vi "Read CarWash Controller Constants.vi"(8 "error in":errorcluster, 11 "CFG File Refnum in":T2) -> (0 "error out":errorcluster, 3 "CFG File Refnum out":T2)   [LabVIEW 2017]
uses:
  <vilib>/Utility/config.llb/Config Data RefNum.ctl
  Configuration Data.ctl
  Car Wash System Globals.vi
  <vilib>/Utility/config.llb/Read Key (U32).vi
  <vilib>/Utility/error.llb/Error Cluster From Error Code.vi
  <vilib>/ErrorRing/Error Ring.xnode
  <vilib>/Utility/config.llb/NI_LVConfig.lvlib
panel:
  out "Cluster":T1
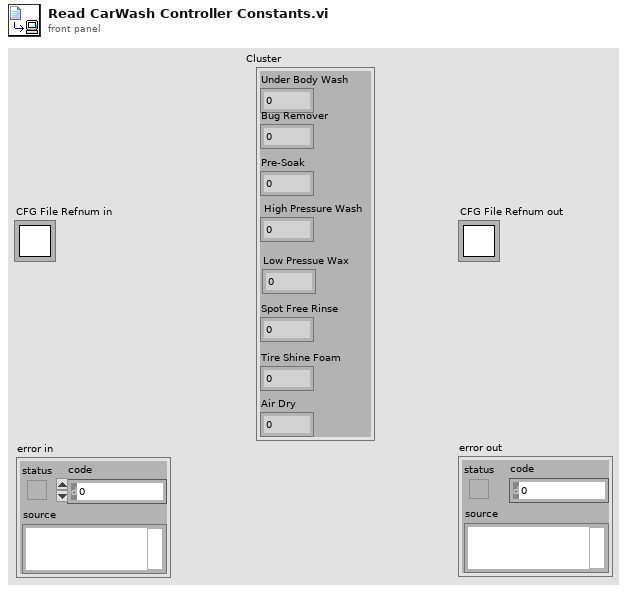
[diagram p1: front panel]
types:
  T1 = typedef "Configuration Data.ctl" = cluster{"Under Body Wash ":u32, "Bug Remover":u32, "Pre-Soak":u32, " High Pressure Wash":u32, "Low Pressue Wax ":u32, "Spot Free Rinse ":u32, "Tire Shine Foam":u32, "Air Dry ":u32}
  T2 = typedef "NI_LVConfig.lvlib/Config Data RefNum.ctl" = refnum<k1>
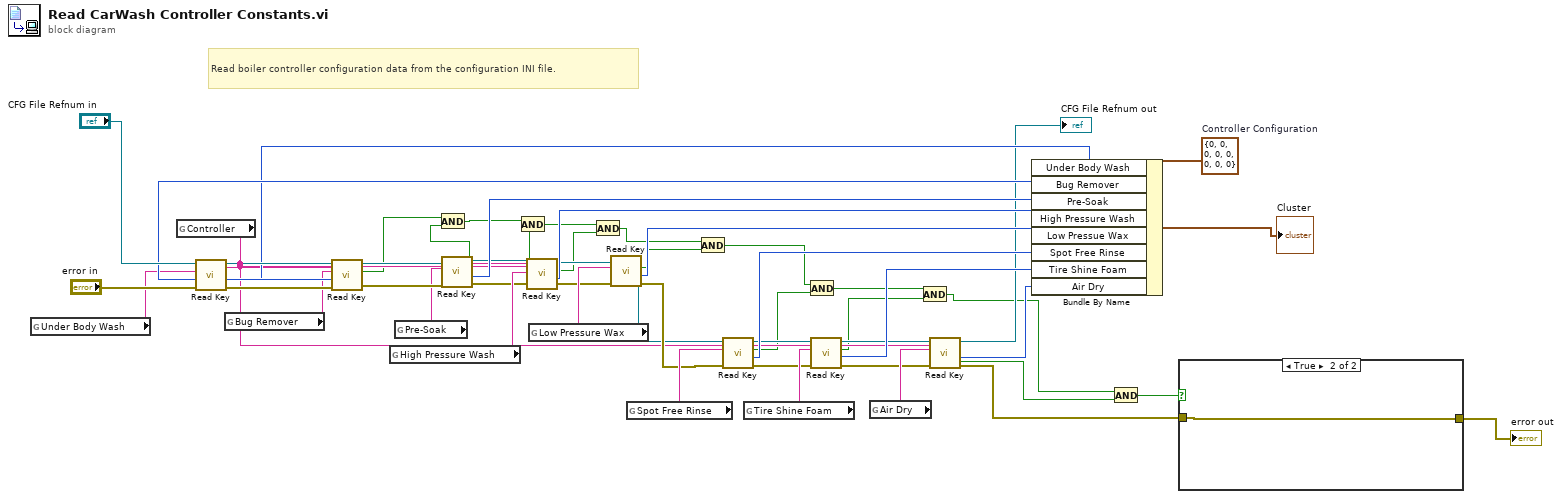
[diagram p0: block diagram]
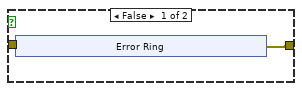
[diagram p2: hidden frame]
diagram:
  w44 = T1 {"Under Body Wash "=0, "Bug Remover"=0, "Pre-Soak"=0, " High Pressure Wash"=0, "Low Pressue Wax "=0, "Spot Free Rinse "=0, "Tire Shine Foam"=0, "Air Dry "=0}  # Controller Configuration
  # "Read boiler controller configuration data from the configuration INI file."
  n1 = global read "Car Wash System Globals.vi" "Under Body Wash"() -> (w46:string)
  n2 = global read "Car Wash System Globals.vi" "Controller"() -> (w19:string)
  n3 = call-poly <vilib>:"Read Key.vi"("section"=w19, "error in (no error)"="error in", "key"=w46, "refnum"="CFG File Refnum in") -> ("error out"=w49:errorcluster, "value"=w45:u32, "refnum out"=w48:T2)  [unwired: 4 in, 1 out]
  n4 = global read "Car Wash System Globals.vi" "Bug Remover"() -> (w43:string)
  n5 = call-poly <vilib>:"Read Key.vi"("section"=w19, "error in (no error)"=w49, "key"=w43, "refnum"=w48) -> ("error out"=w42:errorcluster, "value"=w47:u32, "found?"=w16:bool, "refnum out"=w38:T2)  [unwired: 4 in]
  n6 = global read "Car Wash System Globals.vi" "High Pressure Wash"() -> (w39:string)
  n7 = global read "Car Wash System Globals.vi" "Pre-Soak"() -> (w41:string)
  n8 = call-poly <vilib>:"Read Key.vi"("section"=w19, "error in (no error)"=w42, "key"=w41, "refnum"=w38) -> ("error out"=w36:errorcluster, "value"=w40:u32, "found?"=w15:bool, "refnum out"=w37:T2)  [unwired: 4 in]
  n9 = And(x=w16, y=w15) -> (x .and. y?=w12:bool)
  n10 = call-poly <vilib>:"Read Key.vi"("section"=w19, "error in (no error)"=w36, "key"=w39, "refnum"=w37) -> ("error out"=w32:errorcluster, "value"=w35:u32, "found?"=w13:bool, "refnum out"=w33:T2)  [unwired: 4 in]
  n11 = And(x=w12, y=w13) -> (x .and. y?=w14:bool)
  n12 = global read "Car Wash System Globals.vi" "Low Pressure Wax"() -> (w34:string)
  n13 = And(x=w14, y=w13) -> (x .and. y?=w11:bool)
  n14 = call-poly <vilib>:"Read Key.vi"("section"=w19, "error in (no error)"=w32, "key"=w34, "refnum"=w33) -> ("error out"=w29:errorcluster, "value"=w31:u32, "found?"=w10:bool, "refnum out"=w28:T2)  [unwired: 4 in]
  n15 = global read "Car Wash System Globals.vi" "Spot Free Rinse"() -> (w30:string)
  n16 = And(x=w11, y=w10) -> (x .and. y?=w9:bool)
  n17 = call-poly <vilib>:"Read Key.vi"("section"=w19, "error in (no error)"=w29, "key"=w30, "refnum"=w28) -> ("error out"=w25:errorcluster, "value"=w27:u32, "found?"=w8:bool, "refnum out"=w23:T2)  [unwired: 4 in]
  n18 = global read "Car Wash System Globals.vi" "Tire Shine Foam"() -> (w26:string)
  n19 = And(x=w9, y=w8) -> (x .and. y?=w7:bool)
  n20 = call-poly <vilib>:"Read Key.vi"("section"=w19, "error in (no error)"=w25, "key"=w26, "refnum"=w23) -> ("error out"=w21:errorcluster, "value"=w24:u32, "found?"=w6:bool, "refnum out"=w20:T2)  [unwired: 4 in]
  n21 = global read "Car Wash System Globals.vi" "Air Dry"() -> (w22:string)
  n22 = And(x=w7, y=w6) -> (x .and. y?=w4:bool)
  n23 = call-poly <vilib>:"Read Key.vi"("section"=w19, "error in (no error)"=w21, "key"=w22, "refnum"=w20) -> ("error out"=w2:errorcluster, "value"=w18:u32, "found?"=w5:bool, "refnum out"=→"CFG File Refnum out":T2)  [unwired: 4 in]
  n24 = Bundle By Name(cluster=w44, "Under Body Wash"=w45, "Bug Remover"=w47, "Pre-Soak"=w40, "High Pressure Wash"=w35, "Low Pressue Wax"=w31, "Spot Free Rinse"=w27, "Tire Shine Foam"=w24, "Air Dry"=w18) -> (→"Cluster":T1)
  n25 = And(x=w4, y=w5) -> (x .and. y?=w3:bool)
  n26 = case shown="True" w3 {
    tunnel: [w53 w59] -> w52
    tunnel: w2 -> [_ w59]
    frame False {
      n27 = xnode "Error Ring"() -> ("error out"=w53:errorcluster)
    }
    frame True {
    }
  }
  "error out" <- w52
